vi "Write Variant Value.vi"(7 "Value Type":T1, 8 "error in (no error)":errorcluster, 10 "Value":variant, 11 "Config Element in":refnum<class "Config Element.lvclass">) -> (0 "error out":errorcluster, 3 "Config Element out":refnum<class "Config Element.lvclass">)   [LabVIEW 2023, in "CDM-Config.lvlib" / "Config Element.lvclass"]
uses:
  Config Element.lvclass
  Value Type.ctl
  Config Element.lvclass/Config Element.ctl
  CDM-Config.lvlib
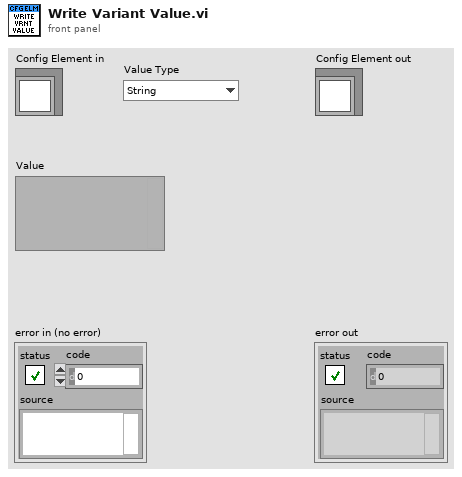
[diagram p1: front panel]
types:
  T1 = typedef "CDM-Config.lvlib/Value Type.ctl" = enum16{"String", "Number", "Bool", "Object", "Array"}
  T2 = typedef "CDM-Config.lvlib/Config Element.lvclass/Element Data.ctl" = cluster{"Node Info":T3, "Owner":refnum<class>, "Changed":bool, "Name":string, "Meta Data":T4[], "Value Type":T1, "Value":variant}
  T3 = typedef "CDM-Config.lvlib/Node Info.ctl" = cluster{"Index":i32, "Parent":i32, "Children":i32[]}
  T4 = typedef "CDM-Config.lvlib/Meta Data.ctl" = cluster{"Name":string, "Value":string}
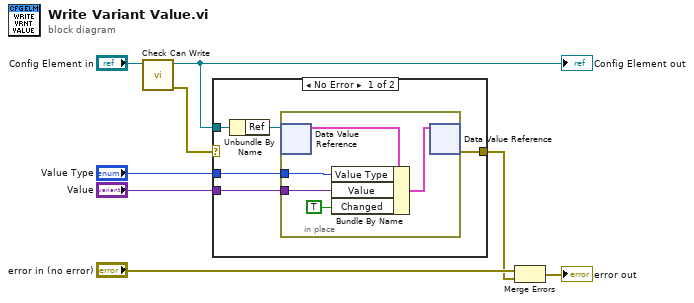
[diagram p0: block diagram]
diagram:
  n1 = call "Check Can Write.vi"("Config Element in"="Config Element in") -> ("error out"=w1:errorcluster, "Config Element out"=w2:refnum<class "Config Element.lvclass">)  [unwired: 9 in]
  "Config Element out" <- w2
  n2 = case shown="No Error" w1 {
    selector: w1 -> [_ w19]
    tunnel: "Value Type" -> [w12 _]
    tunnel: "Value" -> [w11 _]
    tunnel: [w10 w19] -> w3
    tunnel: w2 -> [w9 _]
    frame No Error {
      n3 = Unbundle By Name(w9) -> ("Ref"=w13:refnum<data-value>)
      n4 = in-place {
        in-place-border: w12 -> [w16]
        in-place-border: w11 -> [w15]
        n5 = in-place-dvr #1(w13) -> (w18:T2)  [unwired: 1 out]
        n6 = Bundle By Name(cluster=w18, "Value Type"=w16, "Value"=w15, "Changed"=TRUE) -> (w17:T2)
        n7 = in-place-dvr #1(w17) -> (w10:errorcluster)  [unwired: 1 out]
      }
    }
    frame Error {
    }
  }
  n8 = Merge Errors("error in (no error)", w3) -> (→"error out":errorcluster)
